vi "Supply_ComplianceCheck.vi"(8 "error in (no error)":errorcluster, 11 "KE2657A in":refnum<class "KE2657A.lvclass">) -> (0 "error out":errorcluster, 1 "Status string":string, 2 "Compliance exceeded?":bool, 3 "KE2657A out":refnum<class "KE2657A.lvclass">)   [LabVIEW 2018, in "KE2657A.lvclass"]
uses:
  KE2657A.lvclass
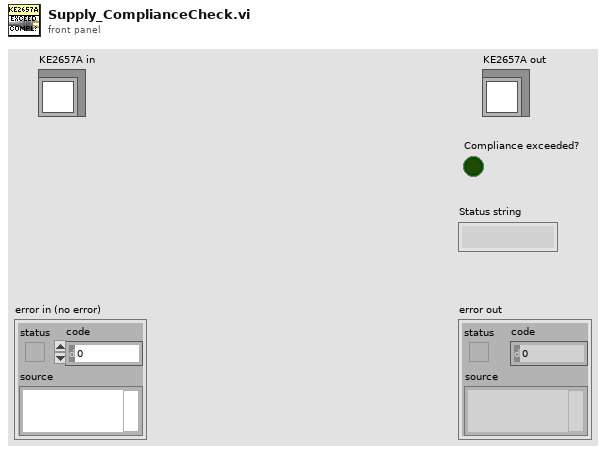
[diagram p1: front panel]
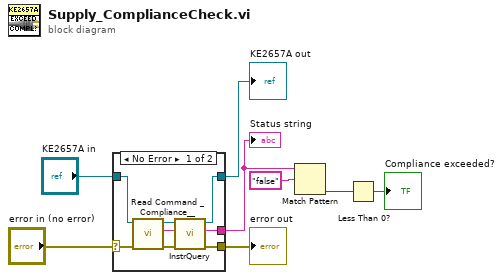
[diagram p0: block diagram]
diagram:
  n1 = case shown="No Error" "error in (no error)" {
    selector: "error in (no error)" -> [w9 w17]
    tunnel: [w16 w17] -> w8
    tunnel: [w15 w18] -> w7
    tunnel: "KE2657A in" -> [w11 w18]
    tunnel: [w10 _] -> w2
    frame No Error {
      n2 = call-dynamic "Read Command _Compliance__.vi"("error in (no error)"=w9, "SupplyControl in"=w11) -> ("error out"=w14:errorcluster, "Command \"Compliance?\""=w13:string, "SupplyControl out"=w12:refnum<class "KE2657A.lvclass">)  [unwired: 7 in]
      n3 = call-dynamic "InstrQuery.vi"("error in (no error)"=w14, "Command string"=w13, "InstControl in"=w12) -> ("error out"=w16:errorcluster, "Instrument response"=w10:string, "InstControl out"=w15:refnum<class "KE2657A.lvclass">)  [unwired: 6 in]
    }
    frame Error {
    }
  }
  "KE2657A out" <- w7
  "error out" <- w8
  "Status string" <- w2
  n4 = Match Pattern(string=w2, regular expression="false") -> (offset past match=w3:i32)  [unwired: 1 in, 3 out]
  n5 = Less Than 0?(x=w3) -> (x < 0?=→"Compliance exceeded?":bool)
